vi "Set Global StateType Filter.vi"(10 "Group:LogType":T1[](array[typedef]), 11 "GlobalLogFilter In":refnum<class "LogFilter.lvclass">) -> (3 "GlobalLogFilter Out":refnum<class "LogFilter.lvclass">)   [LabVIEW 2017, in "Communicable State Machine.lvlib" / "LogFilter.lvclass"]
doc: "### Set Global StateType Filter.vi\n\n-- <b>Controls</b> --\n- <b>Group:LogType</b>:\n- <b>GlobalLogFilter in</b>:\n\n-- <b>Indicators</b> --\n- <b>GlobalLogFilter out</b>:"
uses:
  LogFilter.lvclass
  Typedef/_CSM_GlobalLog_STATE_TYPE.ctl
  LogFilter.lvclass/LogFilter.ctl
  Communicable State Machine.lvlib
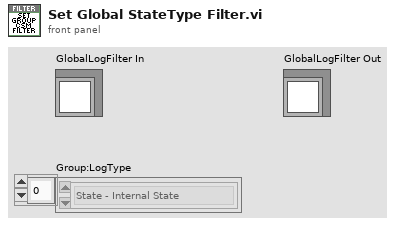
[diagram p1: front panel]
types:
  T1 = typedef "Communicable State Machine.lvlib/_CSM_GlobalLog_STATE_TYPE.ctl" = enum16{"State - Internal State", "State - External Message", "State - Response", "State - Complete"}
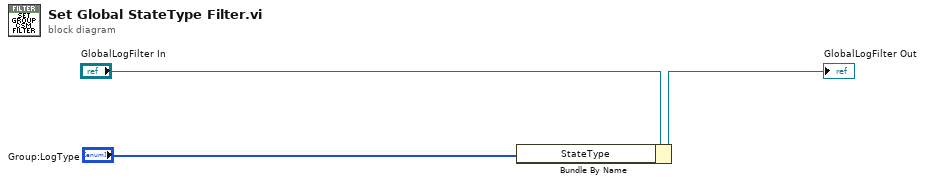
[diagram p0: block diagram]
diagram:
  n1 = Bundle By Name(cluster="GlobalLogFilter In", "StateType"="Group:LogType") -> (→"GlobalLogFilter Out":refnum<class "LogFilter.lvclass">)
